vi "Input_Commands_Conveyor.vi"(11 "All Joysticks":T2) -> (3 "Conveyor Command Inputs":T1)   [LabVIEW 2012]
uses:
  Input_All_Joysticks.ctl
  Input_Single_Joystick.ctl
  <vilib>/Rock Robotics/WPI/Joystick/WPI_JoystickButtonState.ctl
  Input_Command_Conveyor.ctl
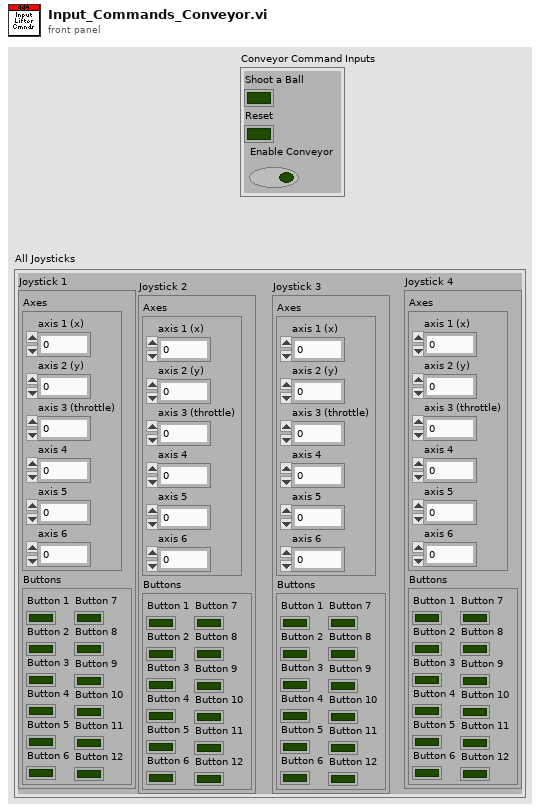
[diagram p1: front panel]
types:
  T1 = typedef "Input_Command_Conveyor.ctl" = cluster{"Shoot a Ball":bool, "Reset":bool, "Enable Conveyor":bool}
  T2 = typedef "Input_All_Joysticks.ctl" = cluster{"Joystick 1":T3, "Joystick 2":T3, "Joystick 3":T3, "Joystick 4":T3}
  T3 = typedef "Input_Single_Joystick.ctl" = cluster{"Axes":cluster{"axis 1 (x)":dbl, "axis 2 (y)":dbl, "axis 3 (throttle)":dbl, "axis 4":dbl, "axis 5":dbl, "axis 6":dbl}, "Buttons":T4}
  T4 = typedef "WPI_JoystickButtonState.ctl" = cluster{"Button 1":bool, "Button 2":bool, "Button 3":bool, "Button 4":bool, "Button 5":bool, "Button 6":bool, "Button 7":bool, "Button 8":bool, "Button 9":bool, "Button 10":bool, "Button 11":bool, "Button 12":bool}
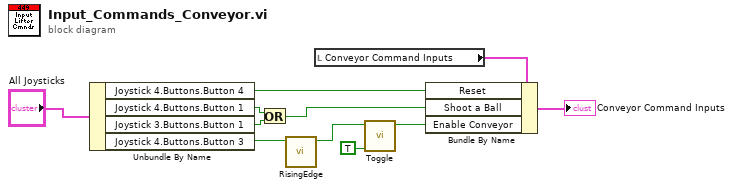
[diagram p0: block diagram]
diagram:
  n1 = Unbundle By Name("All Joysticks") -> ("Joystick 4.Buttons.Button 4"=w10:bool, "Joystick 4.Buttons.Button 1"=w2:bool, "Joystick 3.Buttons.Button 1"=w3:bool, "Joystick 4.Buttons.Button 3"=w5:bool)
  n2 = Or(x=w2, y=w3) -> (x .or. y?=w1:bool)
  n3 = call "RisingEdge.vi"("BooleanIn"=w5) -> ("BooleanOut"=w4:bool)  [unwired: 10 in]
  n4 = local read "Conveyor Command Inputs"() -> (w11:T1)
  n5 = call "Toggle.vi"("Initial"=TRUE, "Toggle"=w4) -> ("BoolOut"=w6:bool)  [unwired: 9 in]
  n6 = Bundle By Name(cluster=w11, "Reset"=w10, "Shoot a Ball"=w1, "Enable Conveyor"=w6) -> (→"Conveyor Command Inputs":T1)
